vi "Arduino New Log File Path.vi"() -> (3 "log ref":refnum<file>)   [LabVIEW 2024, in "FW Arduino Control.lvclass"]
uses:
  FW Arduino Control.lvclass
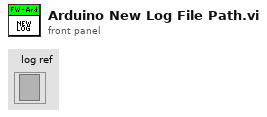
[diagram p1: front panel]
types:
  T1 = enum16{"open", "replace", "create", "open or create", "replace or create", "replace or create with confirmation"}
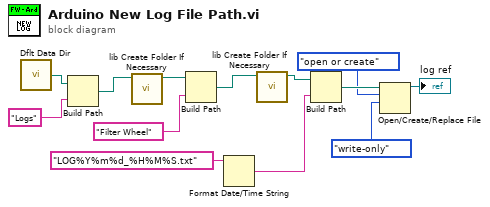
[diagram p0: block diagram]
diagram:
  n1 = call <vilib>:"Dflt Data Dir.vi"() -> ("App:Default Data Directory"=w13:path)
  n2 = Build Path(base path=w13, name or relative path="Logs") -> (appended path=w11:path)
  n3 = call "lib Create Folder If Necessary.vi"("Folder"=w11) -> ("Folder dup"=w10:path)  [unwired: 9 in, 1 out]
  n4 = Build Path(base path=w10, name or relative path="Filter Wheel") -> (appended path=w8:path)
  n5 = Format Date/Time String(time format string (%c)="LOG%Y%m%d_%H%M%S.txt") -> (date/time string=w5:string)  [unwired: 2 in]
  n6 = call "lib Create Folder If Necessary.vi"("Folder"=w8) -> ("Folder dup"=w6:path)  [unwired: 9 in, 1 out]
  n7 = Build Path(base path=w6, name or relative path=w5) -> (appended path=w4:path)
  n8 = Open/Create/Replace File(file path (use dialog)=w4, operation (0:open)=T1."open or create", access (0:read/write)=enum16{"read/write", "read-only", "write-only"}."write-only") -> (refnum out=→"log ref":refnum<file>)  [unwired: 3 in, 2 out]
